vi "Server_Training.vi"(8 "error in":errorcluster, 11 "Main Update Data":T1) -> (0 "error out":errorcluster)   [LabVIEW 2018, in "Cloud Server.lvlib"]
uses:
  Cloud Server.lvlib
  Data Def/Server_Main Update Data.ctl
  Data Def/Server_Connection Manager Method.ctl
  Data Def/Server_Training Data.ctl
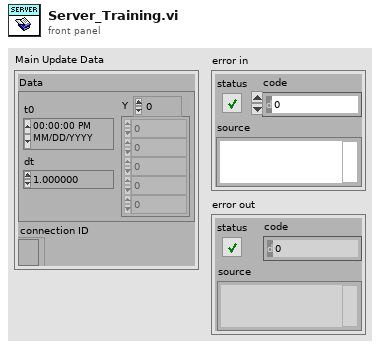
[diagram p1: front panel]
types:
  T1 = typedef "Cloud Server.lvlib/Server_Main Update Data.ctl" = cluster{"Data":waveform(dbl), "connection ID":refnum<k5>}
  T2 = typedef "Cloud Server.lvlib/Server_Connection Manager Method.ctl" = enum16{"Initialize", "Add", "Get", "Set Properties", "Get Properties", "Close", "Release"}
  T3 = typedef "Cloud Server.lvlib/Server_Connection Properties.ctl" = cluster{"User Data":T4, "Data":waveform(dbl)}
  T4 = typedef "User Data.ctl" = cluster{"Name":string, "Email":string, "Phone Number":string, "User Picture":u32[][], "Last Login Time":timestamp}
  T5 = typedef "Cloud Server.lvlib/Server_Training Data.ctl" = cluster{"Data":waveform(dbl), "Abnormal?":bool}
  T6 = enum16{"open", "replace", "create", "open or create", "replace or create", "replace or create with confirmation"}
  T7 = typedef "Cloud Server.lvlib/Server_Main Data.ctl" = cluster{"Main VI Ref.":refnum<vi>, "Listener ID":refnum<k5>, "Meta data":T8[], "Main Queue":T10, "User Picture":T11}
  T8 = typedef "stm_MetaElement.ctl" = cluster{"Name":T9}
  T9 = typedef "stm_MetaDataElement.ctl" = string
  T10 = typedef "Cloud Server.lvlib/Server_Main Queue.ctl" = cluster{"Server Write Queue":refnum<queue>, "Main Loop Queue":refnum<queue>}
  T11 = typedef "IMAQ Image.ctl" = refnum<image>
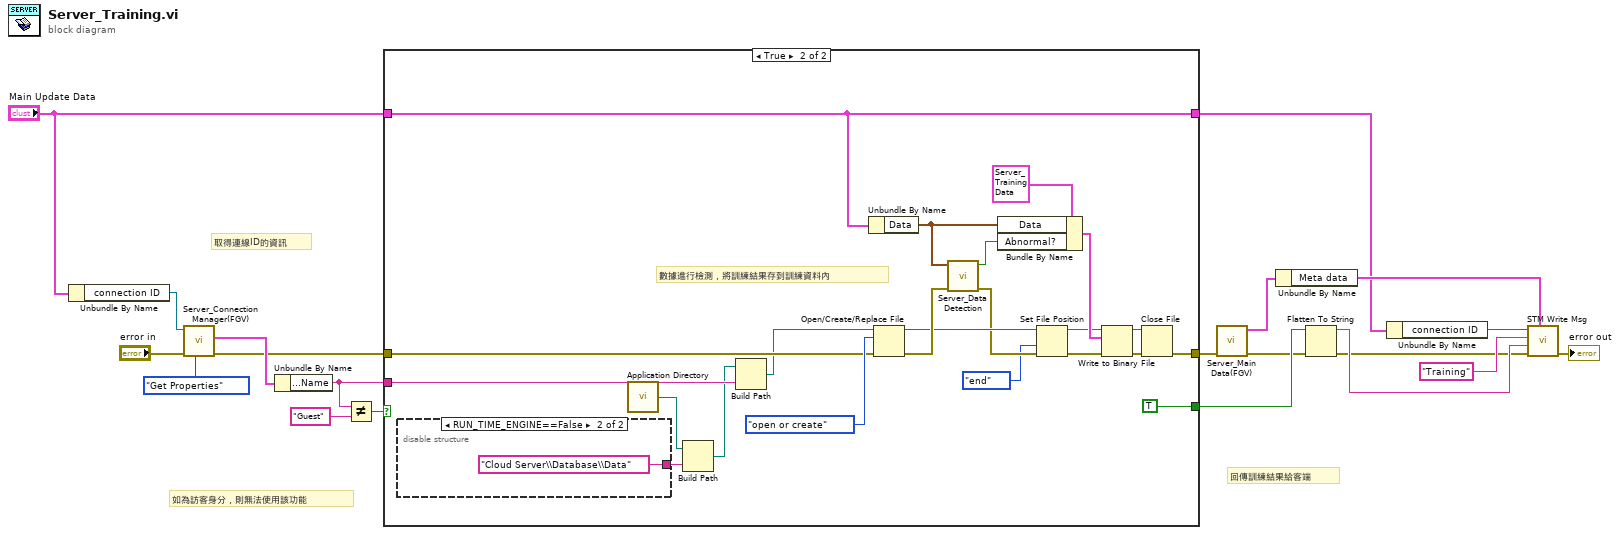
[diagram p0: block diagram]
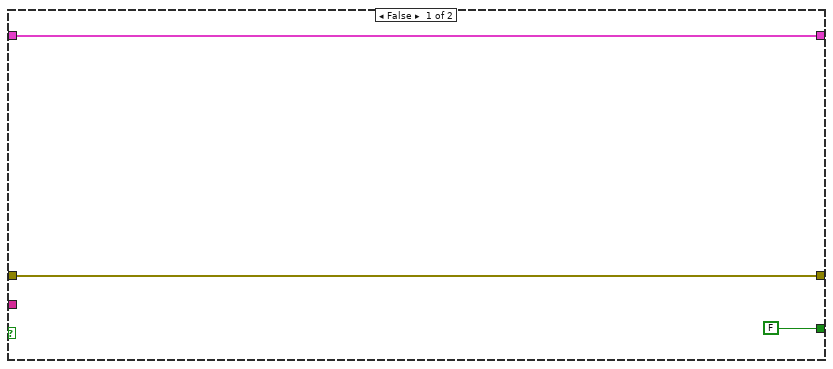
[diagram p2: hidden frame]
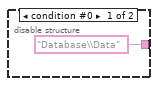
[diagram p3: hidden frame]
diagram:
  # "回傳訓練結果給客端"
  # "如為訪客身分，則無法使用該功能"
  # "取得連線ID的資訊"
  n1 = Unbundle By Name("Main Update Data") -> ("connection ID"=w18:refnum<k5>)
  n2 = call "Server_Connection Manager(FGV).vi"("Connection Manager Method(Get)"=Server_Connection_Manager_Method."Get Properties", "error in"="error in", "Connection In"=w18) -> ("error out"=w12:errorcluster, "Connection Properties Out"=w17:T3)  [unwired: 4 in, 3 out]
  n3 = Unbundle By Name(w17) -> ("User Data.Name"=w13:string)
  n4 = Not Equal?(x=w13, y="Guest" ("x")) -> (x != y?=w15:bool)
  n5 = case shown="True" w15 {
    tunnel: "Main Update Data" -> [w22 w37]
    tunnel: w12 -> [w23 w34]
    tunnel: [w23 w38] -> w3
    tunnel: w13 -> [_ w43]
    tunnel: [w22 w37] -> w6
    tunnel: [FALSE TRUE] -> w5
    frame False {
    }
    frame True {
      # "數據進行檢測，將訓練結果存到訓練資料內"
      n6 = disable-structure shown="RUN_TIME_ENGINE==False" {
        disable-tunnel: ["Database\\Data" ("name or relative path") "Cloud Server\\Database\\Data" ("name or relative path")] -> w45
        frame condition #0 {
        }
        frame condition #1 (active) {
        }
      }
      n7 = call <vilib>:"Application Directory.vi"() -> ("Application Directory"=w44:path)
      n8 = Build Path(base path=w44, name or relative path=w45) -> (appended path=w42:path)
      n9 = Build Path(base path=w42, name or relative path=w43) -> (appended path=w33:path)
      n10 = Unbundle By Name(w37) -> ("Data"=w31:waveform(dbl))
      n11 = Open/Create/Replace File(file path (use dialog)=w33, error in=w34, operation (0:open)=T6."open or create") -> (refnum out=w26:refnum<file>, error out=w41:errorcluster)  [unwired: 3 in, 1 out]
      n12 = call "Server_Data Detection.vi"("error in"=w41, "Data"=w31) -> ("error out"=w25:errorcluster, "Warning?"=w30:bool)  [unwired: 8 in]
      n13 = Bundle By Name(cluster=T5 {"Data"={"t0"=timestamp(0 s since 1904-01-01), "dt"=1.0, "Y"=[]}, "Abnormal?"=FALSE} ("Training Data"), "Data"=w31, "Abnormal?"=w30) -> (w29:T5)
      n14 = Set File Position(refnum=w26, from (0:start)=enum16{"start", "end", "current"}."end", error in=w25) -> (refnum out=w28:refnum<file>, error out=w27:errorcluster)  [unwired: 1 in]
      n15 = Write to Binary File(file (use dialog)=w28, data=w29, error in=w27) -> (refnum out=w39:refnum<file>, error out=w40:errorcluster)  [unwired: 3 in, 1 out]
      n16 = Close File(refnum=w39, error in=w40) -> (error out=w38:errorcluster)  [unwired: 1 out]
    }
  }
  n17 = call "Server_Main Data(FGV).vi"("error in"=w3) -> ("error out"=w2:errorcluster, "Main Data Out"=w1:T7)  [unwired: 9 in]
  n18 = Unbundle By Name(w1) -> ("Meta data"=w7:T8[])
  n19 = Flatten To String(anything=w5, error in (no error)=w2) -> (data string=w11:string, error out=w9:errorcluster)  [unwired: 2 in, 1 out]
  n20 = Unbundle By Name(w6) -> ("connection ID"=w8:refnum<k5>)
  n21 = call "STM Write Msg.vi"("Meta data"=w7, "error in (no error)"=w9, "Data"=w11, "Name"="Training", "connection ID"=w8) -> ("error out"=→"error out":errorcluster)  [unwired: 5 in, 1 out]
